vi "Remove Graphic Object.vi"(8 "error in (no error)":errorcluster, 10 "ID":i32, 11 "Canvas in":refnum<class "Canvas.lvclass">) -> (0 "error out":errorcluster, 3 "Canvas out":refnum<class "Canvas.lvclass">)   [LabVIEW 2015, in "Canvas.lvclass"]
uses:
  Canvas.lvclass
  Canvas.lvclass/Canvas.ctl
  Graphic/Graphic.lvclass/Graphic.ctl
  Graphic/Graphic.lvclass
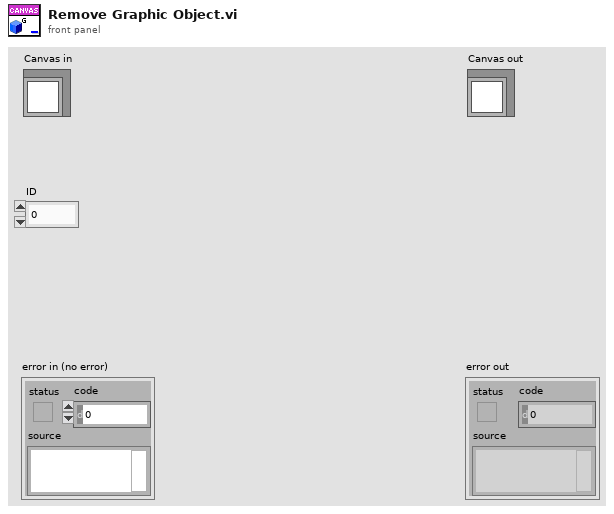
[diagram p1: front panel]
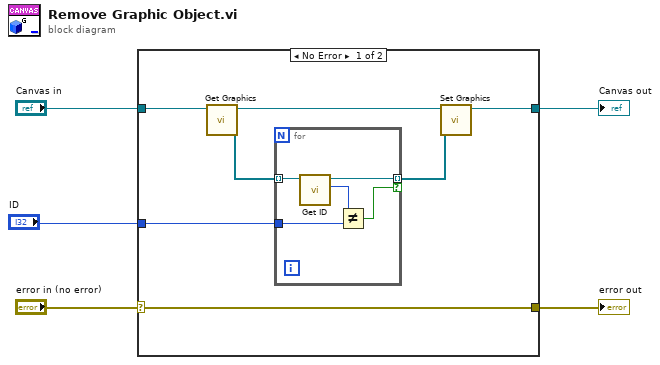
[diagram p0: block diagram]
diagram:
  n1 = case shown="No Error" "error in (no error)" {
    selector: "error in (no error)" -> [w11 w19]
    tunnel: [w11 w19] -> w4
    tunnel: [w7 w18] -> w2
    tunnel: "Canvas in" -> [w12 w18]
    tunnel: "ID" -> [w8 _]
    frame No Error {
      n2 = call "Get Graphics.vi"("Canvas in"=w12) -> ("Graphics"=w9:refnum<class "Graphic.lvclass">[], "Canvas out"=w10:refnum<class "Canvas.lvclass">)  [unwired: 8 in, 1 out]
      n3 = for {
        tunnel: w9 -> [w17] mode=indexing
        tunnel: [w16] -> w6 mode=indexing if=w13
        tunnel: w8 -> [w14]
        n4 = call "Get ID.vi"("Graphic in"=w17) -> ("ID"=w15:i32, "Graphic out"=w16:refnum<class "Graphic.lvclass">)  [unwired: 8 in, 1 out]
        n5 = Not Equal?(x=w15, y=w14) -> (x != y?=w13:bool)
      }
      n6 = call "Set Graphics.vi"("Graphics"=w6, "Canvas in"=w10) -> ("Canvas out"=w7:refnum<class "Canvas.lvclass">)  [unwired: 8 in, 1 out]
    }
    frame Error {
    }
  }
  "error out" <- w4
  "Canvas out" <- w2
